vi "Path to Data Type.vi"(8 "error in (no error)":errorcluster, 11 "Path":path) -> (0 "error out":errorcluster, 3 "Boolean out":refnum<class "Path.lvclass">)   [LabVIEW 2017, in "Path.lvclass"]
uses:
  <vilib>/gpm_packages/@cs/data-type-serializer/source/Path/Path.lvclass
  <vilib>/gpm_packages/@cs/data-type-serializer/source/Path/Path.lvclass/Path.ctl
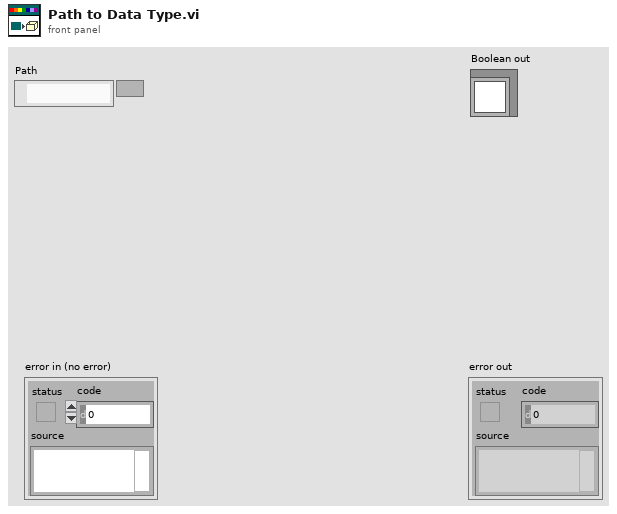
[diagram p1: front panel]
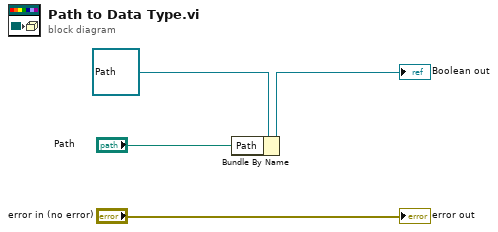
[diagram p0: block diagram]
diagram:
  n1 = Bundle By Name(cluster=refnum<class "Path.lvclass"> refnum ("Boolean in"), "Path"="Path") -> (→"Boolean out":refnum<class "Path.lvclass">)
  "error out" <- "error in (no error)"
